vi "Step Counter.Get Step.vi"(11 "Step State":T1) -> (2 "Cntr":i32, 3 "Step":string)   [LabVIEW 2018]
uses:
  Step Counter.State Info.ctl
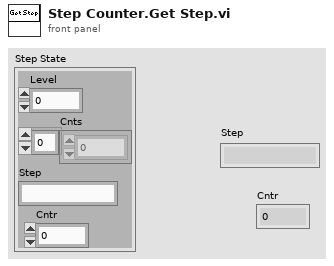
[diagram p1: front panel]
types:
  T1 = typedef "Step Counter.State Info.ctl" = cluster{"Level":i32, "Cnts":i32[], "Step":string, "Cntr":i32}
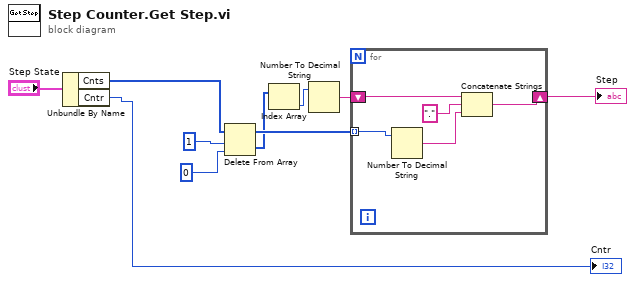
[diagram p0: block diagram]
diagram:
  n1 = Unbundle By Name("Step State") -> ("Cnts"=w10:i32[], "Cntr"=→"Cntr":i32)
  n2 = Delete From Array(array=w10, length=1, index=0) -> (deleted portion=w4:i32[], array with subset deleted=w9:i32[])
  n3 = Index Array(array=w4) -> (element=w5:i32)  [unwired: 1 in]
  n4 = Number To Decimal String(number=w5) -> (decimal integer string=w8:string)  [unwired: 1 in]
  n5 = for {
    tunnel: w9 -> [w13] mode=indexing
    shift-right: [w14] -> w2
    shift-left: w8 -> [w15]
    n6 = Number To Decimal String(number=w13) -> (decimal integer string=w12:string)  [unwired: 1 in]
    n7 = Concatenate Strings(w15, ".", w12) -> (w14:string)
  }
  "Step" <- w2
